vi "Initialize Queues.vi"(8 "error in (no error)":errorcluster, 11 "Work Dispatcher in":refnum<class "Work Dispatcher.lvclass">) -> (0 "error out":errorcluster, 3 "Work Dispatcher out":refnum<class "Work Dispatcher.lvclass">)   [LabVIEW 2020, in "Work Dispatcher.lvclass"]
uses:
  Work Dispatcher.lvclass
  Work Dispatcher.lvclass/Work Dispatcher.ctl
  People/Process Job/Job Handler.lvclass
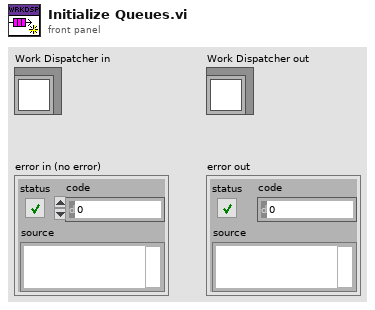
[diagram p1: front panel]
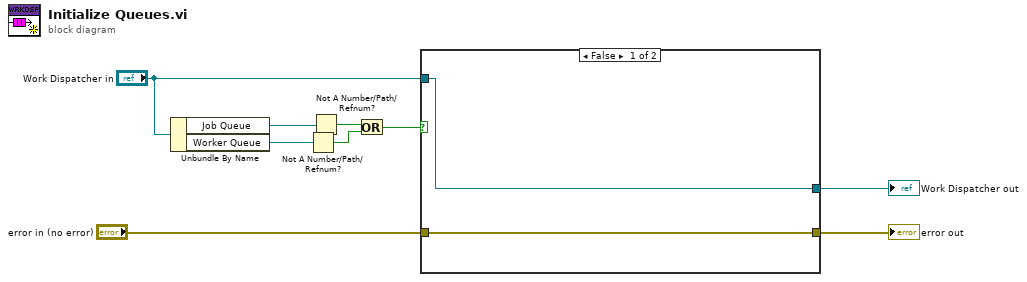
[diagram p0: block diagram]
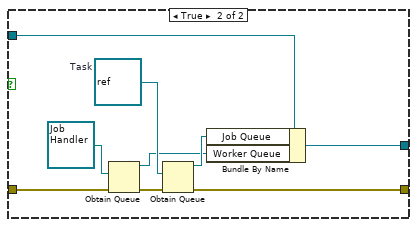
[diagram p2: hidden frame]
diagram:
  n1 = Unbundle By Name("Work Dispatcher in") -> ("Job Queue"=w5:refnum<queue>, "Worker Queue"=w4:refnum<queue>)
  n2 = Not A Number/Path/Refnum?(number/path/refnum=w4) -> (NaN/Path/Refnum?=w2:bool)
  n3 = Not A Number/Path/Refnum?(number/path/refnum=w5) -> (NaN/Path/Refnum?=w3:bool)
  n4 = Or(x=w3, y=w2) -> (x .or. y?=w1:bool)
  n5 = case shown="False" w1 {
    tunnel: [w11 w19] -> w9
    tunnel: [w10 w17] -> w8
    tunnel: "error in (no error)" -> [w10 w15]
    tunnel: "Work Dispatcher in" -> [w11 w12]
    frame False {
    }
    frame True {
      w18 = refnum<class> refnum  # Task
      n6 = Obtain Queue(element data type=refnum<class "Job Handler.lvclass"> refnum ("Process Job.lvclass"), error in (no error)=w15) -> (queue out=w13:refnum<queue>, error out=w16:errorcluster)  [unwired: 3 in, 1 out]
      n7 = Obtain Queue(element data type=w18, error in (no error)=w16) -> (queue out=w20:refnum<queue>, error out=w17:errorcluster)  [unwired: 3 in, 1 out]
      n8 = Bundle By Name(cluster=w12, "Job Queue"=w20, "Worker Queue"=w13) -> (w19:refnum<class "Work Dispatcher.lvclass">)
    }
  }
  "Work Dispatcher out" <- w9
  "error out" <- w8
